vi "Get Data.vi"(0 "Dataset name":string, 1 "Date range":bool, 2 "Record count":bool, 3 "Record Limit":i32, 5 "error in (no error)":errorcluster, 6 "START DATE":timestamp format="%<%.0X %x>T", 7 "Template":string, 8 "END DATE":timestamp format="%<%.0X %x>T", 10 "Date Column":string) -> (14 "data":string[][](array[string]), 19 "error out":errorcluster)   [LabVIEW 2020]
uses:
  <vilib>/addons/database/Connection.llb/Conn ObjectReference.ctl
  <vilib>/addons/database/Connection.llb/DB Tools Open Connec (String).vi
  <vilib>/addons/database/Connection.llb/DB Tools Open Connec (Path).vi
  <vilib>/addons/database/Connection.llb/Conn Execute.vi
  <vilib>/addons/database/Recordset.llb/Rec Fetch Recordset Data (R).vi
  <vilib>/addons/database/Recordset.llb/Rec Destroy - Connection.vi
  <vilib>/addons/database/_DB Variant To Data/Database Variant To Data.xnode
  <vilib>/addons/database/NI_Database_API.lvlib
panel:
  out "String":string
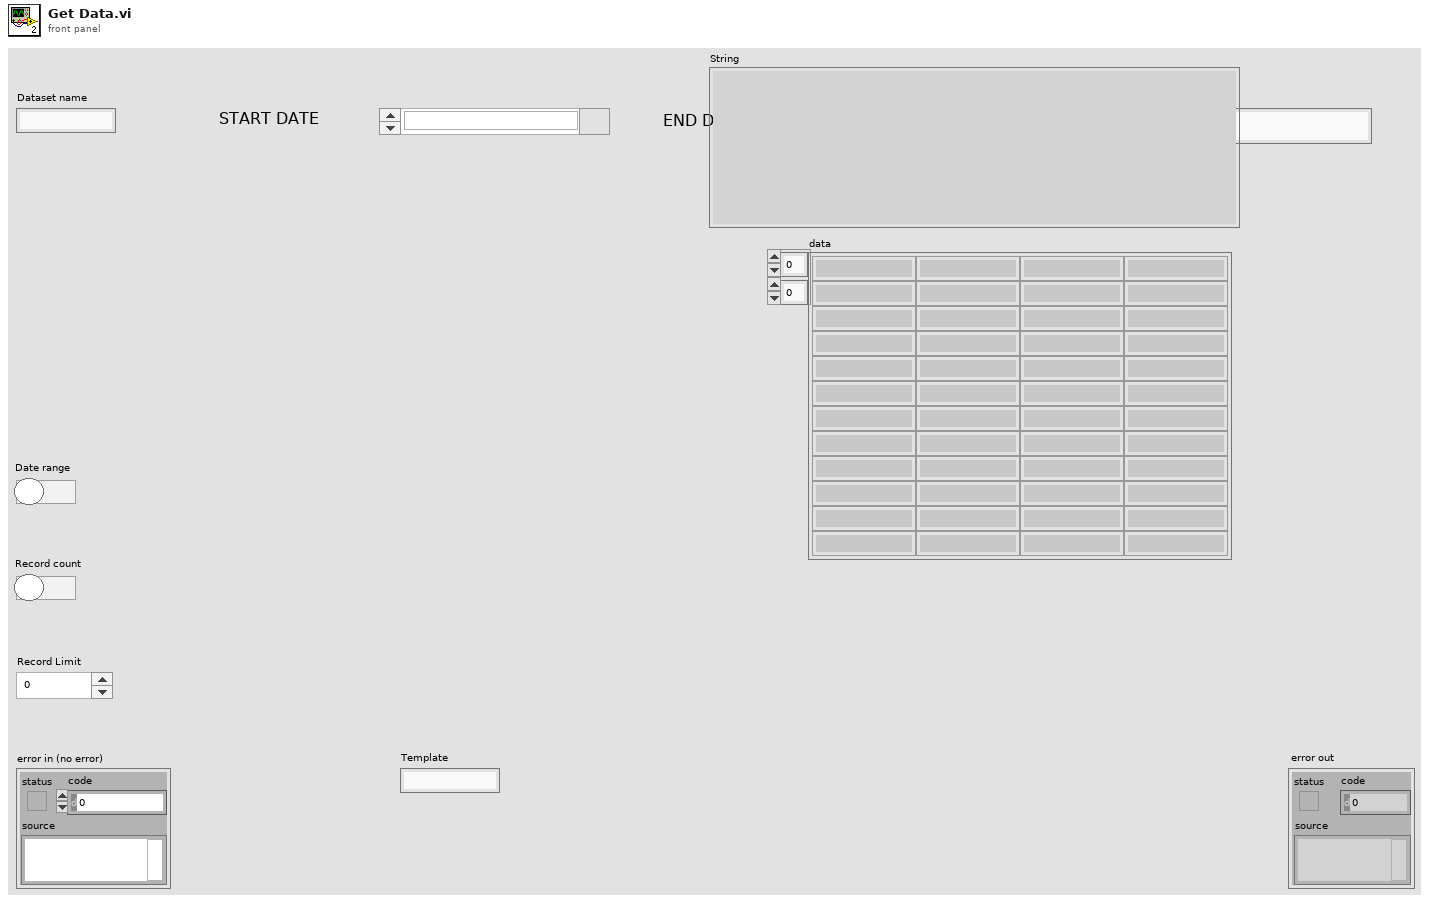
[diagram p1: front panel]
types:
  T1 = cluster{"Query":string, "DB Type":string, "Data Source name":string}
  T2 = typedef "Connection Information.ctl" = cluster{"Username":string, "Password":string, "Server Address":string, "Port":u32, "Schema Name":string, "Driver":string, "Connection String":string, "Data Source Name":string, "Database Selector":string, "ULD FIle or Connection String":bool, "UDL Path":path}
  T3 = typedef "Config Cluster.ctl" = cluster{"MYSQL":cluster{"SHOW DATABASE":string, "SHOW TABLES":string, "SHOW COLUMNS":string}, "SQL Server":cluster{"SHOW DATABASE":string, "SHOW TABLES":string, "SHOW COLUMNS":string}}
  T4 = typedef "NI_Database_API.lvlib/Conn ObjectReference.ctl" = refnum<k1>
  T5 = typedef "NI_Database_API.lvlib/Rec ObjectReference.ctl" = refnum<k1>
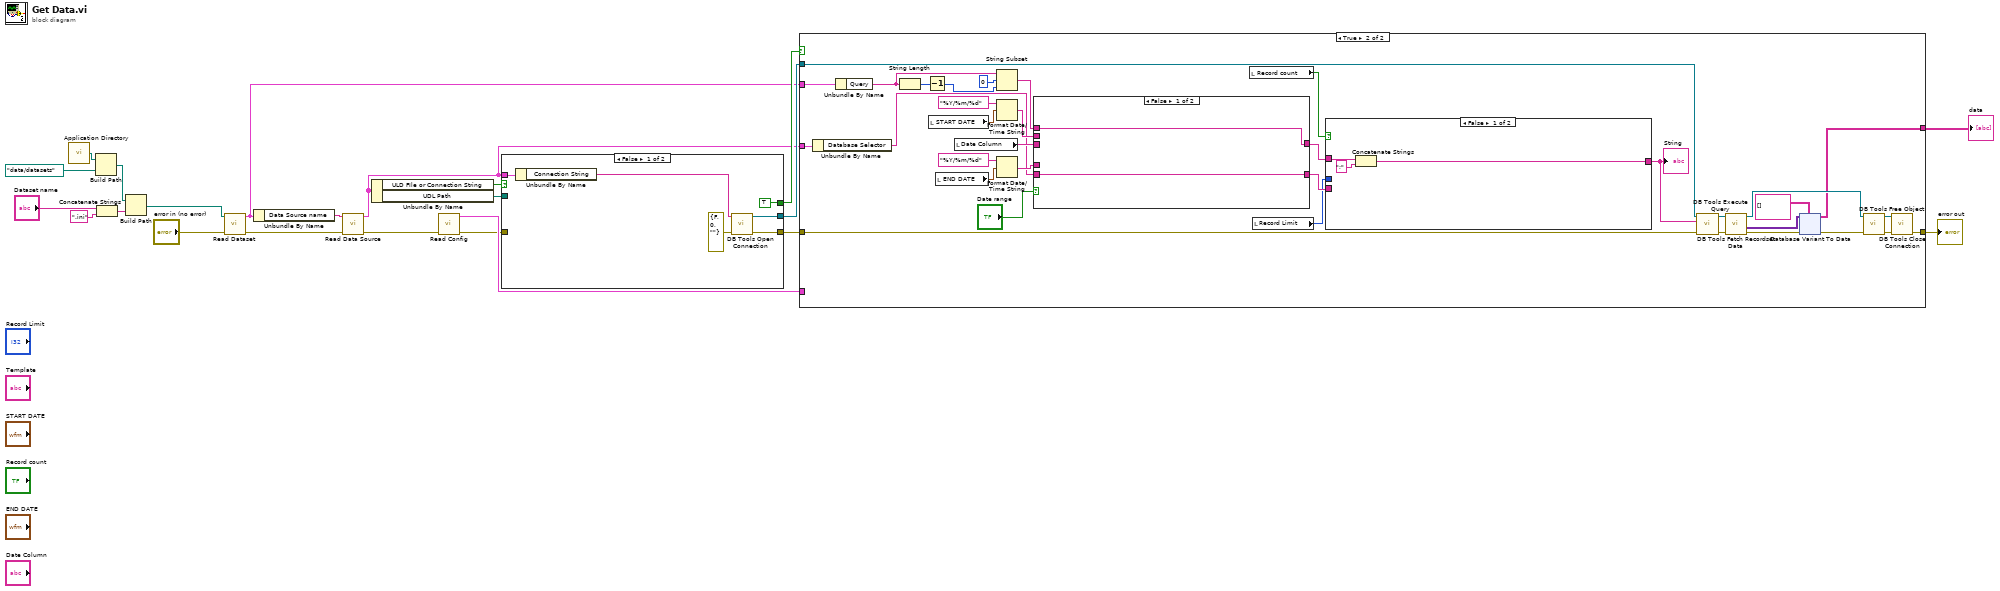
[diagram p0: block diagram]
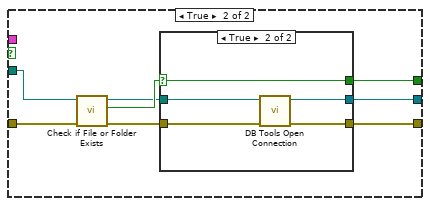
[diagram p2: hidden frame]
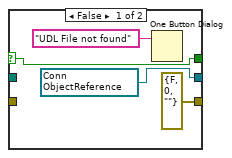
[diagram p3: hidden frame]
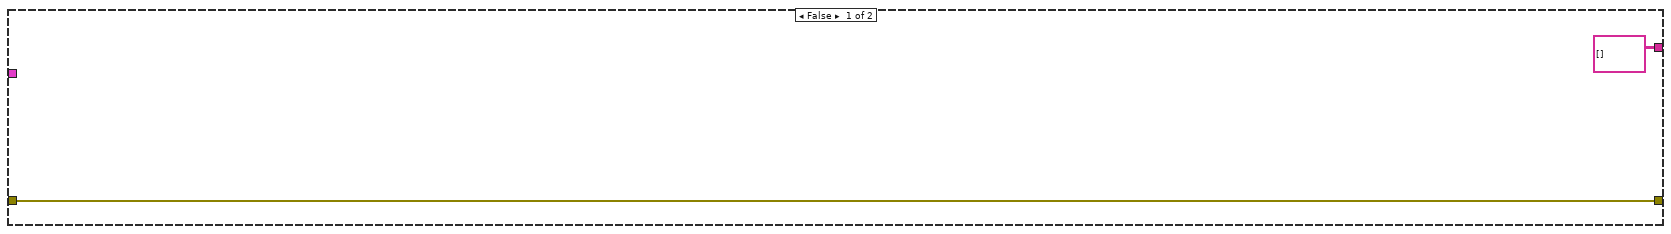
[diagram p4: hidden frame]
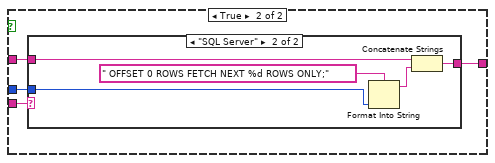
[diagram p5: hidden frame]
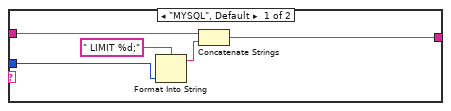
[diagram p6: hidden frame]
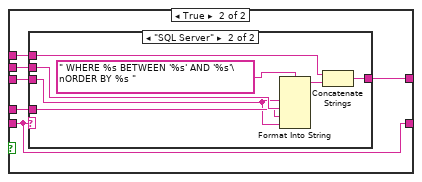
[diagram p7: hidden frame]
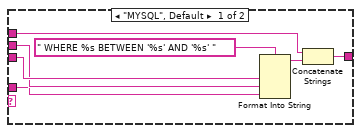
[diagram p8: hidden frame]
diagram:
  n1 = call <vilib>:"Application Directory.vi"() -> ("Application Directory"=w10:path)
  n2 = Build Path(base path=w10, name or relative path=path "data/datasets") -> (appended path=w8:path)
  n3 = Concatenate Strings("Dataset name", ".ini" ("string")) -> (w4:string)
  n4 = Build Path(base path=w8, name or relative path=w4) -> (appended path=w7:path)
  n5 = call "Read Dataset.vi"("error in (no error)"="error in (no error)", "Saving Path"=w7) -> ("error out"=w11:errorcluster, "Information"=w5:T1)  [unwired: 8 in]
  n6 = Unbundle By Name(w5) -> ("Data Source name"=w12:string)
  n7 = call "Read Data Source.vi"("error in (no error)"=w11, "Data Source Name"=w12) -> ("error out"=w22:errorcluster, "Connection Information"=w15:T2)  [unwired: 8 in]
  n8 = Unbundle By Name(w15) -> ("ULD FIle or Connection String"=w20:bool, "UDL Path"=w19:path)
  n9 = call "Read Config.vi"("error in (no error)"=w22) -> ("error out"=w6:errorcluster, "Config"=w21:T3)  [unwired: 9 in]
  n10 = case shown="False" w20 {
    tunnel: w19 -> [_ w36]
    tunnel: [TRUE ("file or folder exists?") w34] -> w18
    tunnel: [w26 w30] -> w17
    tunnel: [w25 w31] -> w16
    tunnel: w15 -> [w24 _]
    tunnel: w6 -> [_ w29]
    frame False {
      n11 = Unbundle By Name(w24) -> ("Connection String"=w23:string)
      n12 = call-poly <vilib>:"DB Tools Open Connection.vi"("error in (no error)"=errorcluster {"status"=FALSE, "code"=0, "source"=""} ("error out"), "connection information"=w23) -> ("error out"=w26:errorcluster, "connection reference"=w25:T4)  [unwired: 6 in]
    }
    frame True {
      n13 = call <vilib>:"Check if File or Folder Exists.vi"("error in (no error)"=w29, "path"=w36) -> ("error out"=w32:errorcluster, "file or folder exists?"=w35:bool, "dup path"=w33:path)  [unwired: 7 in]
      n14 = case shown="True" w35 {
        selector: w35 -> [w39 w45]
        tunnel: [w39 w45] -> w34
        tunnel: w33 -> [_ w44]
        tunnel: w32 -> [_ w43]
        tunnel: [w38 w42] -> w31
        tunnel: [errorcluster {"status"=FALSE, "code"=0, "source"=""} ("error out") w41] -> w30
        frame False {
          w38 = T4 refnum items=["Connection"] ("connection reference")
          n15 = One Button Dialog(message="UDL File not found") -> ()  [unwired: 1 in, 1 out]
        }
        frame True {
          n16 = call-poly <vilib>:"DB Tools Open Connection.vi"("error in (no error)"=w43, "connection information"=w44) -> ("error out"=w41:errorcluster, "connection reference"=w42:T4)  [unwired: 6 in]
        }
      }
    }
  }
  n17 = case shown="True" w18 {
    tunnel: w15 -> [_ w71]
    tunnel: w17 -> [w47 w73]
    tunnel: w16 -> [_ w72]
    tunnel: w21 -> [_ _]
    tunnel: [w47 w70] -> w14
    tunnel: w5 -> [_ w68]
    tunnel: [string[][] [] ("data") w48] -> w1
    frame False {
    }
    frame True {
      n18 = Unbundle By Name(w71) -> ("Database Selector"=w54:string)
      n19 = Unbundle By Name(w68) -> ("Query"=w63:string)
      n20 = String Length(string=w63) -> (length=w65:i32)
      n21 = Decrement(x=w65) -> (x-1=w66:i32)
      n22 = local read "START DATE"() -> (w60:timestamp)
      n23 = local read "END DATE"() -> (w56:timestamp)
      n24 = local read "Date Column"() -> (w61:string)
      n25 = String Subset(string=w63, offset (0)=0, length (rest)=w66) -> (substring=w62:string)
      n26 = Format Date/Time String(time format string (%c)="%Y/%m/%d", seconds (now)=w60) -> (date/time string=w58:string)  [unwired: 1 in]
      n27 = Format Date/Time String(time format string (%c)="%Y/%m/%d", seconds (now)=w56) -> (date/time string=w55:string)  [unwired: 1 in]
      n28 = case shown="False" "Date range" {
        tunnel: w62 -> [w100 w106]
        tunnel: [w100 w102] -> w53
        tunnel: w61 -> [_ w105]
        tunnel: w58 -> [_ w104]
        tunnel: w55 -> [_ w103]
        tunnel: w54 -> [w99 w101]
        tunnel: [w99 w101] -> w51
        frame False {
        }
        frame True {
          n29 = case shown="\"SQL Server\"" w101 {
            tunnel: w106 -> [w112 w115]
            tunnel: w105 -> [w110 w117]
            tunnel: w104 -> [w109 w119]
            tunnel: w103 -> [w108 w118]
            tunnel: [w107 w114] -> w102
            frame "MYSQL", Default {
              n30 = Format Into String(format string=" WHERE %s BETWEEN '%s' AND '%s' ", w110, w109, w108) -> (resulting string=w111:string)  [unwired: 2 in, 1 out]
              n31 = Concatenate Strings(w112, w111) -> (w107:string)
            }
            frame "SQL Server" {
              n32 = Format Into String(format string=" WHERE %s BETWEEN '%s' AND '%s'\nORDER BY %s ", w117, w119, w118, w117) -> (resulting string=w116:string)  [unwired: 2 in, 1 out]
              n33 = Concatenate Strings(w115, w116) -> (w114:string)
            }
          }
        }
      }
      n34 = local read "Record count"() -> (w52:bool)
      n35 = local read "Record Limit"() -> (w50:i32)
      n36 = case shown="False" w52 {
        tunnel: w53 -> [w84 w87]
        tunnel: w51 -> [_ w88]
        tunnel: w50 -> [_ w86]
        tunnel: [w82 w85] -> w49
        frame False {
          n37 = Concatenate Strings(w84, ";" ("string")) -> (w82:string)
        }
        frame True {
          n38 = case shown="\"SQL Server\"" w88 {
            tunnel: [w91 w96] -> w85
            tunnel: w87 -> [w90 w95]
            tunnel: w86 -> [w89 w94]
            frame "MYSQL", Default {
              n39 = Format Into String(format string=" LIMIT %d;", w89) -> (resulting string=w92:string)  [unwired: 2 in, 1 out]
              n40 = Concatenate Strings(w90, w92) -> (w91:string)
            }
            frame "SQL Server" {
              n41 = Format Into String(format string=" OFFSET 0 ROWS FETCH NEXT %d ROWS ONLY;", w94) -> (resulting string=w97:string)  [unwired: 2 in, 1 out]
              n42 = Concatenate Strings(w95, w97) -> (w96:string)
            }
          }
        }
      }
      "String" <- w49
      n43 = call-poly <vilib>:"DB Tools Execute Query.vi"("error in (no error)"=w73, "SQL query"=w49, "connection reference"=w72) -> ("error out"=w80:errorcluster, "recordset reference"=w81:T5)  [unwired: 5 in]
      n44 = call-poly <vilib>:"DB Tools Fetch Recordset Data.vi"("error in (no error)"=w80, "recordset reference"=w81) -> ("error out"=w76:errorcluster, "recordset data"=w78:variant[][], "recordset reference out"=w79:T5)  [unwired: 3 in]
      n45 = xnode "Database Variant To Data"("database variant"=w78, "error in (no error)"=w76, "type"=string[][] []) -> ("data"=w48:string[][], "error out"=w75:errorcluster)
      n46 = call-poly <vilib>:"DB Tools Free Object.vi"("error in (no error)"=w75, "recordset reference"=w79) -> ("error out"=w74:errorcluster, "connection reference"=w69:T4)  [unwired: 8 in]
      n47 = call <vilib>:"DB Tools Close Connection.vi"("error in (no error)"=w74, "connection reference"=w69) -> ("error out"=w70:errorcluster)  [unwired: 5 in]
    }
  }
  "error out" <- w14
  "data" <- w1
